vi "Uart Get Available Bytes.vi"(8 "error in (no error)":errorcluster, 10 "Channel":u8, 11 "LINX Client in":refnum<class "LINX Client.lvclass">) -> (0 "error out":errorcluster, 1 "Num Bytes":i32, 3 "LINX Client out":refnum<class "LINX Client.lvclass">)   [LabVIEW 2020, in "LINX Client.lvclass"]
uses:
  LINX Client.lvclass
  LINX Client.lvclass/LINX Client.ctl
  LINX Base.lvclass
  Z:/Development/LabVIEW Hobbyist Toolkit/LabVIEW/vi.lib/MakerHub/LINX/API/LINX Base.lvclass
  Z:/Development/LabVIEW Hobbyist Toolkit/LabVIEW/vi.lib/MakerHub/LINX/API/LINX Client.lvclass
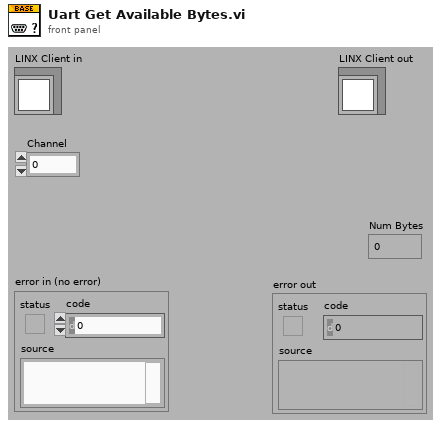
[diagram p1: front panel]
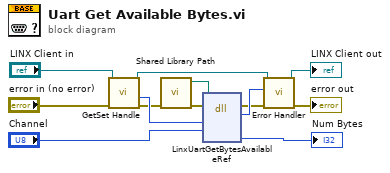
[diagram p0: block diagram]
diagram:
  n1 = call-dynamic "GetSet Handle.vi"("error in"="error in (no error)", "LINX Base in"="LINX Client in") -> ("error out"=w1:errorcluster, "handle out"=w2:u64, "LINX Base out"=w3:refnum<class "LINX Client.lvclass">)  [unwired: 6 in, 1 out]
  n2 = call "Shared Library Path.vi"("error in (no error)"=w1) -> ("error out"=w12:errorcluster, "Path"=w13:path)  [unwired: 9 out]
  n3 = dll-call lib="Z:/Development/LabVIEW Hobbyist Toolkit/LabVIEW/vi.lib/MakerHub/LINX/Resources/libLinxDevice.dll" fn="LinxUartGetBytesAvailableRef"(path in=w13, error in=w12, "device"=w2, "channel"="Channel") -> (error out=w9:errorcluster, "LinxStatus"=w11:i32, "bytes"=→"Num Bytes":i32)  [unwired: 2 in, 3 out]
  n4 = call "Error Handler.vi"("error in (no error)"=w9, "LINX error code"=w11, "LINX Base in"=w3) -> ("error out"=→"error out":errorcluster, "LINX Base out"=→"LINX Client out":refnum<class "LINX Client.lvclass">)  [unwired: 1 in, 6 out]
